vi "Dashboard Main.vi"() -> ()   [LabVIEW 2014]
uses:
  <vilib>/event_ctls.llb/eventvkey.ctl
  <vilib>/Rock Robotics/WPI/Dashboard/WPI_DashboardLogging Global.vi
  <vilib>/Rock Robotics/Network Tables/SD Write String.vi
  <vilib>/Rock Robotics/Network Tables/SD Write Numeric Array.vi
  <vilib>/Utility/config.llb/Write Key (String).vi
  <vilib>/Utility/config.llb/Write Key (I32).vi
  <vilib>/Utility/config.llb/NI_LVConfig.lvlib
panel:
  in  "Close Arm Time":dbl
  in  "TCP":refnum<k5>
  in  "Rec Mode":enum32{"Stop", "Record", "Playback"}(radio)
  in  "Vision":u16(ring) items=["Camera Off", "USB Camera SW", "USB Camera HW", "IP Camera"]
  out "Camera IP":string
  out "Image Message":string="Timeout in Camera Communications"
  in  "Dashboard Tab":T1(tab)
  in  "Camera Settings":T2={"Frame Rate"=30, "Compression"=30, "Size"=1} {"Frame Rate" scale=1.0..30.0; "Size" items=["640x480", "320x240", "160x120"]}
  out "MotorChart R":cluster{"Numeric":dbl, "Numeric":dbl}(graph)
  out "MotorChart L":T3(graph)
  out "MotorSliders R":cluster{"MotorSlide1":dbl, "MotorSlide2":dbl} {"MotorSlide2" scale=-1.0..1.0 scale format="%#_2e"; "MotorSlide1" scale=-1.0..1.0 scale format="%#_2e"}
  out "MotorSliders L":T4 {"MotorSlide4 2" scale=0.0..14.0 scale format="%#_2e"; "MotorSlide2" scale=-1.0..1.0 scale format="%#_2e"; "MotorSlide1" scale=-1.0..1.0 scale format="%#_2e"}
  out "Gyro":dbl(knob) scale=0.0..360.0
  out "JS1 Z":dbl(slide) scale=-1.0..1.0 scale format="%#_2e"
  out "JS1 Graph":cluster{"X":dbl, "Y":dbl}[](graph)
  out "JS1 Buttons":T5
  out "JS2 Z":dbl(slide) scale=-1.0..1.0 scale format="%#_2e"
  out "JS2 Graph":cluster{"X":dbl, "Y":dbl}[](graph)
  out "JS2 Buttons":T5
  out "Mode":T6(ring)=enum."Auto Disabled"
  in  "DB Camera Config":bool
  out "fps":dbl format="%#.1g"
  out "Mbps":dbl format="%#.1g"
  out "Mbps 2":bool
  in  "DB/String 9":string
  in  "DB/String 8":string
  in  "DB/String 7":string
  in  "DB/String 6":string
  in  "DB/String 5":string
  in  "DB/String 4":string
  in  "DB/String 3":string
  in  "DB/String 2":string
  in  "DB/String 1":string
  in  "DB/String 0":string
  in  "DB/Slider 0":dbl(slide) scale=0.0..5.0
  in  "DB/Slider 1":dbl(slide) scale=0.0..5.0
  in  "DB/Slider 2":dbl(slide) scale=0.0..5.0
  in  "DB/Slider 3":dbl(slide) scale=0.0..5.0
  out "DB/LED 3":bool
  out "DB/LED 2":bool
  out "DB/LED 1":bool
  out "DB/LED 0":bool
  in  "DB/Button 3":bool
  in  "DB/Button 2":bool
  in  "DB/Button 1":bool
  in  "DB/Button 0":bool caption="New Name"
  in  "Auto Mode":string(combo)
  in  "Slidewheel Speed":dbl
  in  "Desired Arm Speed":dbl
  in  "Drive Speed":dbl
  in  "Desired Arm Stop":dbl
  in  "Desired Stop Distance":dbl
  in  "Test Slider":dbl(slide) scale=0.0..100.0 scale format="%#_3g"
  in  "On/Off":bool caption="Solenoid"
  in  "Test Name":u16(ring) items=["Select the test to run...", "Example Test", "-------------------------------", "List of tests is built in robot code.", "Replace with your own automated tests."]
  in  "Test Tree":string(tree)
  in  "Motor":cluster{"Value":dbl, "Enable":bool} {"Value" scale=-1.0..1.0 scale format="%#_3g"}
  out "Progress":T7 {"Test Progress" scale=0.0..100.0}
  in  "Rev/Fwd":cluster{"Forward":bool, "Reverse":bool}
  in  "Test Ring":u16(ring) items=["Monochrome", "Color"]
  in  "Listbox":i32(listbox)
  out "Tree":string(tree)
  out "Camera Image":T8(plugin-control)
  out "Boolean":bool
  # "Left"
  # "Front"
  # "Right"
  # "Battery"
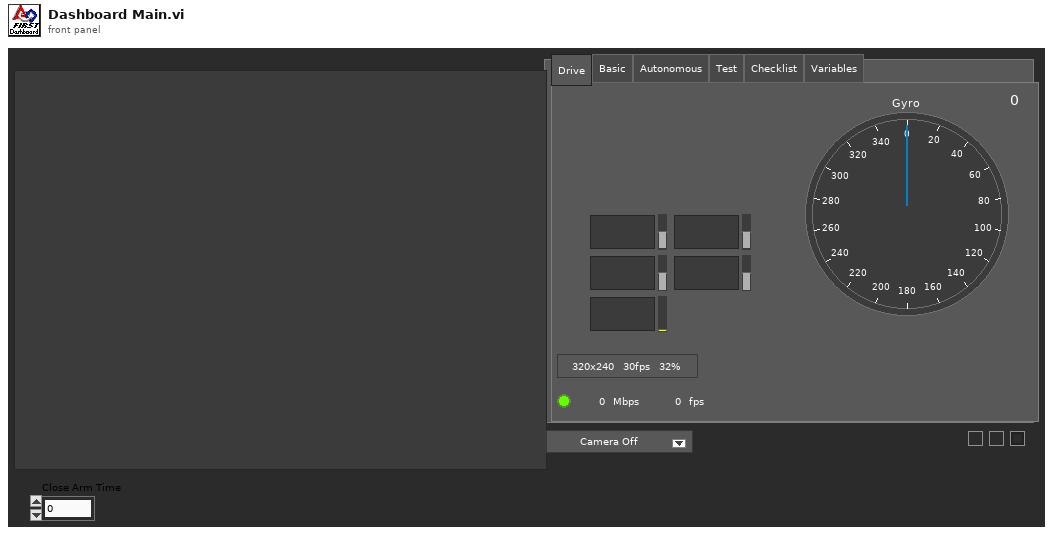
[diagram p1: front panel]
types:
  T1 = enum32{"Drive", "Basic", "Autonomous", "Test", "Checklist", "Variables"}
  T2 = cluster{"Frame Rate":i32, "Compression":i32, "Size":u16}
  T3 = cluster{"Numeric":dbl, "Numeric":dbl, "Battery V":dbl}
  T4 = cluster{"MotorSlide1":dbl, "MotorSlide2":dbl, "MotorSlide4 2":dbl}
  T5 = cluster{bool, bool, bool, bool, bool, bool, bool, bool, bool, bool, bool, bool}
  T6 = enum8{"Tele-Op Disabled", "Tele-Op Enabled", "Auto Disabled", "Auto Enabled", "Test Disabled", "Test Enabled", "Disconnected", "No Code", "E-Stop"}
  T7 = cluster{"Test Progress":u8, "Test Progress Text":string}
  T8 = typedef "IMAQ Image.ctl" = refnum<image>
  T9 = enum32{"Drive", "Basic", "Custom", "Test", "Checklist", "Variables"}
  T10 = typedef "Image Type" = u32
  T11 = cluster{"Camera Image":refnum<vi>, "Dashboard Tab":refnum<vi>, "Boolean":refnum<vi>, "Vision":refnum<vi>, "Rec Mode":refnum<vi>, "Test Slider":refnum<vi>, "On/Off ":refnum<vi>, "Test Ring":refnum<vi>, "Rev/Fwd":refnum<vi>, "Test Name":refnum<vi>, "Motor":refnum<vi>, "Progress":refnum<vi>, "CheckList":refnum<vi>, "Tree":refnum<vi>, "Test Tree":refnum<vi>}
  T12 = cluster{"Error Strings":string, "Disable Counts":cluster{u16, u16}, "Rail Faults":cluster{u16, u16, u16}, "Robot IP":string, "DB Mode":u8, "Event Info":cluster{"Name":string, "Type":u8, "Number":u16, "Replay":u8}, "Camera Addr":string}
  T13 = cluster{"Storage":cluster{"Disk Free":u64, "RAM Block":u32, "RAM free":u32}, "CPU Utilization":cluster{"CPU % ISR":sgl, "CPU % Time Crit":sgl, "CPU % Timed Str":sgl, "CPU % High":sgl, "CPU % Above":sgl, "CPU % Normal":sgl, "CPU % Low":sgl}, "CAN":cluster{"% Bus Utilization":sgl, "Bus Off Cnt":u32, "TX_FIFO Full Cnt":u32, "Receive Error Cnt":u8, "Transmit Error Cnt":u8}, "HID":cluster{"HID Outputs":u32, "Rumble Low":u16, "Rumble High":u16}[]}
  T14 = cluster{"Status bits":cluster{"Test Mode":bool, "Autonomous":bool, "Enabled":bool, "Code Start":bool, "Brownout":bool, "Reserved 2":bool, "Reserved 3":bool, "E-Stop":bool}, "Code Trace":cluster{"Disabled":bool, "TeleOp":bool, "Auto":bool, "Test":bool}, "Controller Type":enum16{"unknown", "cRIO", "roboRio"}, "Code?":enum16{"unknown", "noCode", "code"}, "Battery V":dbl}
  T15 = cluster{"Control Bits":cluster{"TestMode":bool, "Autonomous":bool, "Enabled":bool, "FMS Present":bool, bool, bool, bool, "E-Stop":bool}, "Team Station ":u8, "Countdown":sgl, "Joystick Values":cluster{"Axes":dbl[], "Buttons":bool[], "POVs":i16[]}[]}
  T16 = cluster{"Axes":dbl[], "Buttons":bool[], "POVs":i16[]}[]
  T17 = cluster{"Axes":dbl[], "Buttons":bool[], "POVs":i16[]}
  T18 = cluster{"Buttons[0]":bool, "Buttons[1]":bool, "Buttons[2]":bool, "Buttons[3]":bool, "Buttons[4]":bool, "Buttons[5]":bool, "Buttons[6]":bool, "Buttons[7]":bool, "Buttons[8]":bool, "Buttons[9]":bool, "Buttons[10]":bool, "Buttons[11]":bool}
  T19 = typedef "NI_LVConfig.lvlib/Config Data RefNum.ctl" = refnum<k1>
  T20 = cluster{"Operation":enum16{"Update", "Clear"}, "Color Box":u32}[]
  T21 = typedef "eventvkey.ctl" = enum16{"ASCII", "Enter", "Return", "Shift", "Ctrl", "Alt", "Cmd", "Opt", "Caps", "NumLock", "Clear", "Break", "Up", "Down", "Left", "Right", "Insert", "Delete", "Home", "End", "PageUp", "PageDown", "Escape", "Help", "Pause", "ScrollLock", "F1", "F2", "F3", "F4", "F5", "F6", "F7", "F8", "F9", "F10", "F11", "F12", "F13", "F14", "F15", "F16", "F17", "F18", "F19", "F20", "F21", "F22", "F23", "F24", "Play", "VolumeUp", "VolumeDown", "Mute", "Two Byte Char"}
  T22 = cluster{"Image Size":bool, "Image Type":bool, "Pixel Value":bool, "ROI Information":bool, "Zoom Factor":bool}
  T23 = enum8{"Enabled", "Disabled", "Disabled and Grayed Out"}
  T24 = cluster{"Operation":enum16{"Update", "Clear"}, "Color Box":u32}
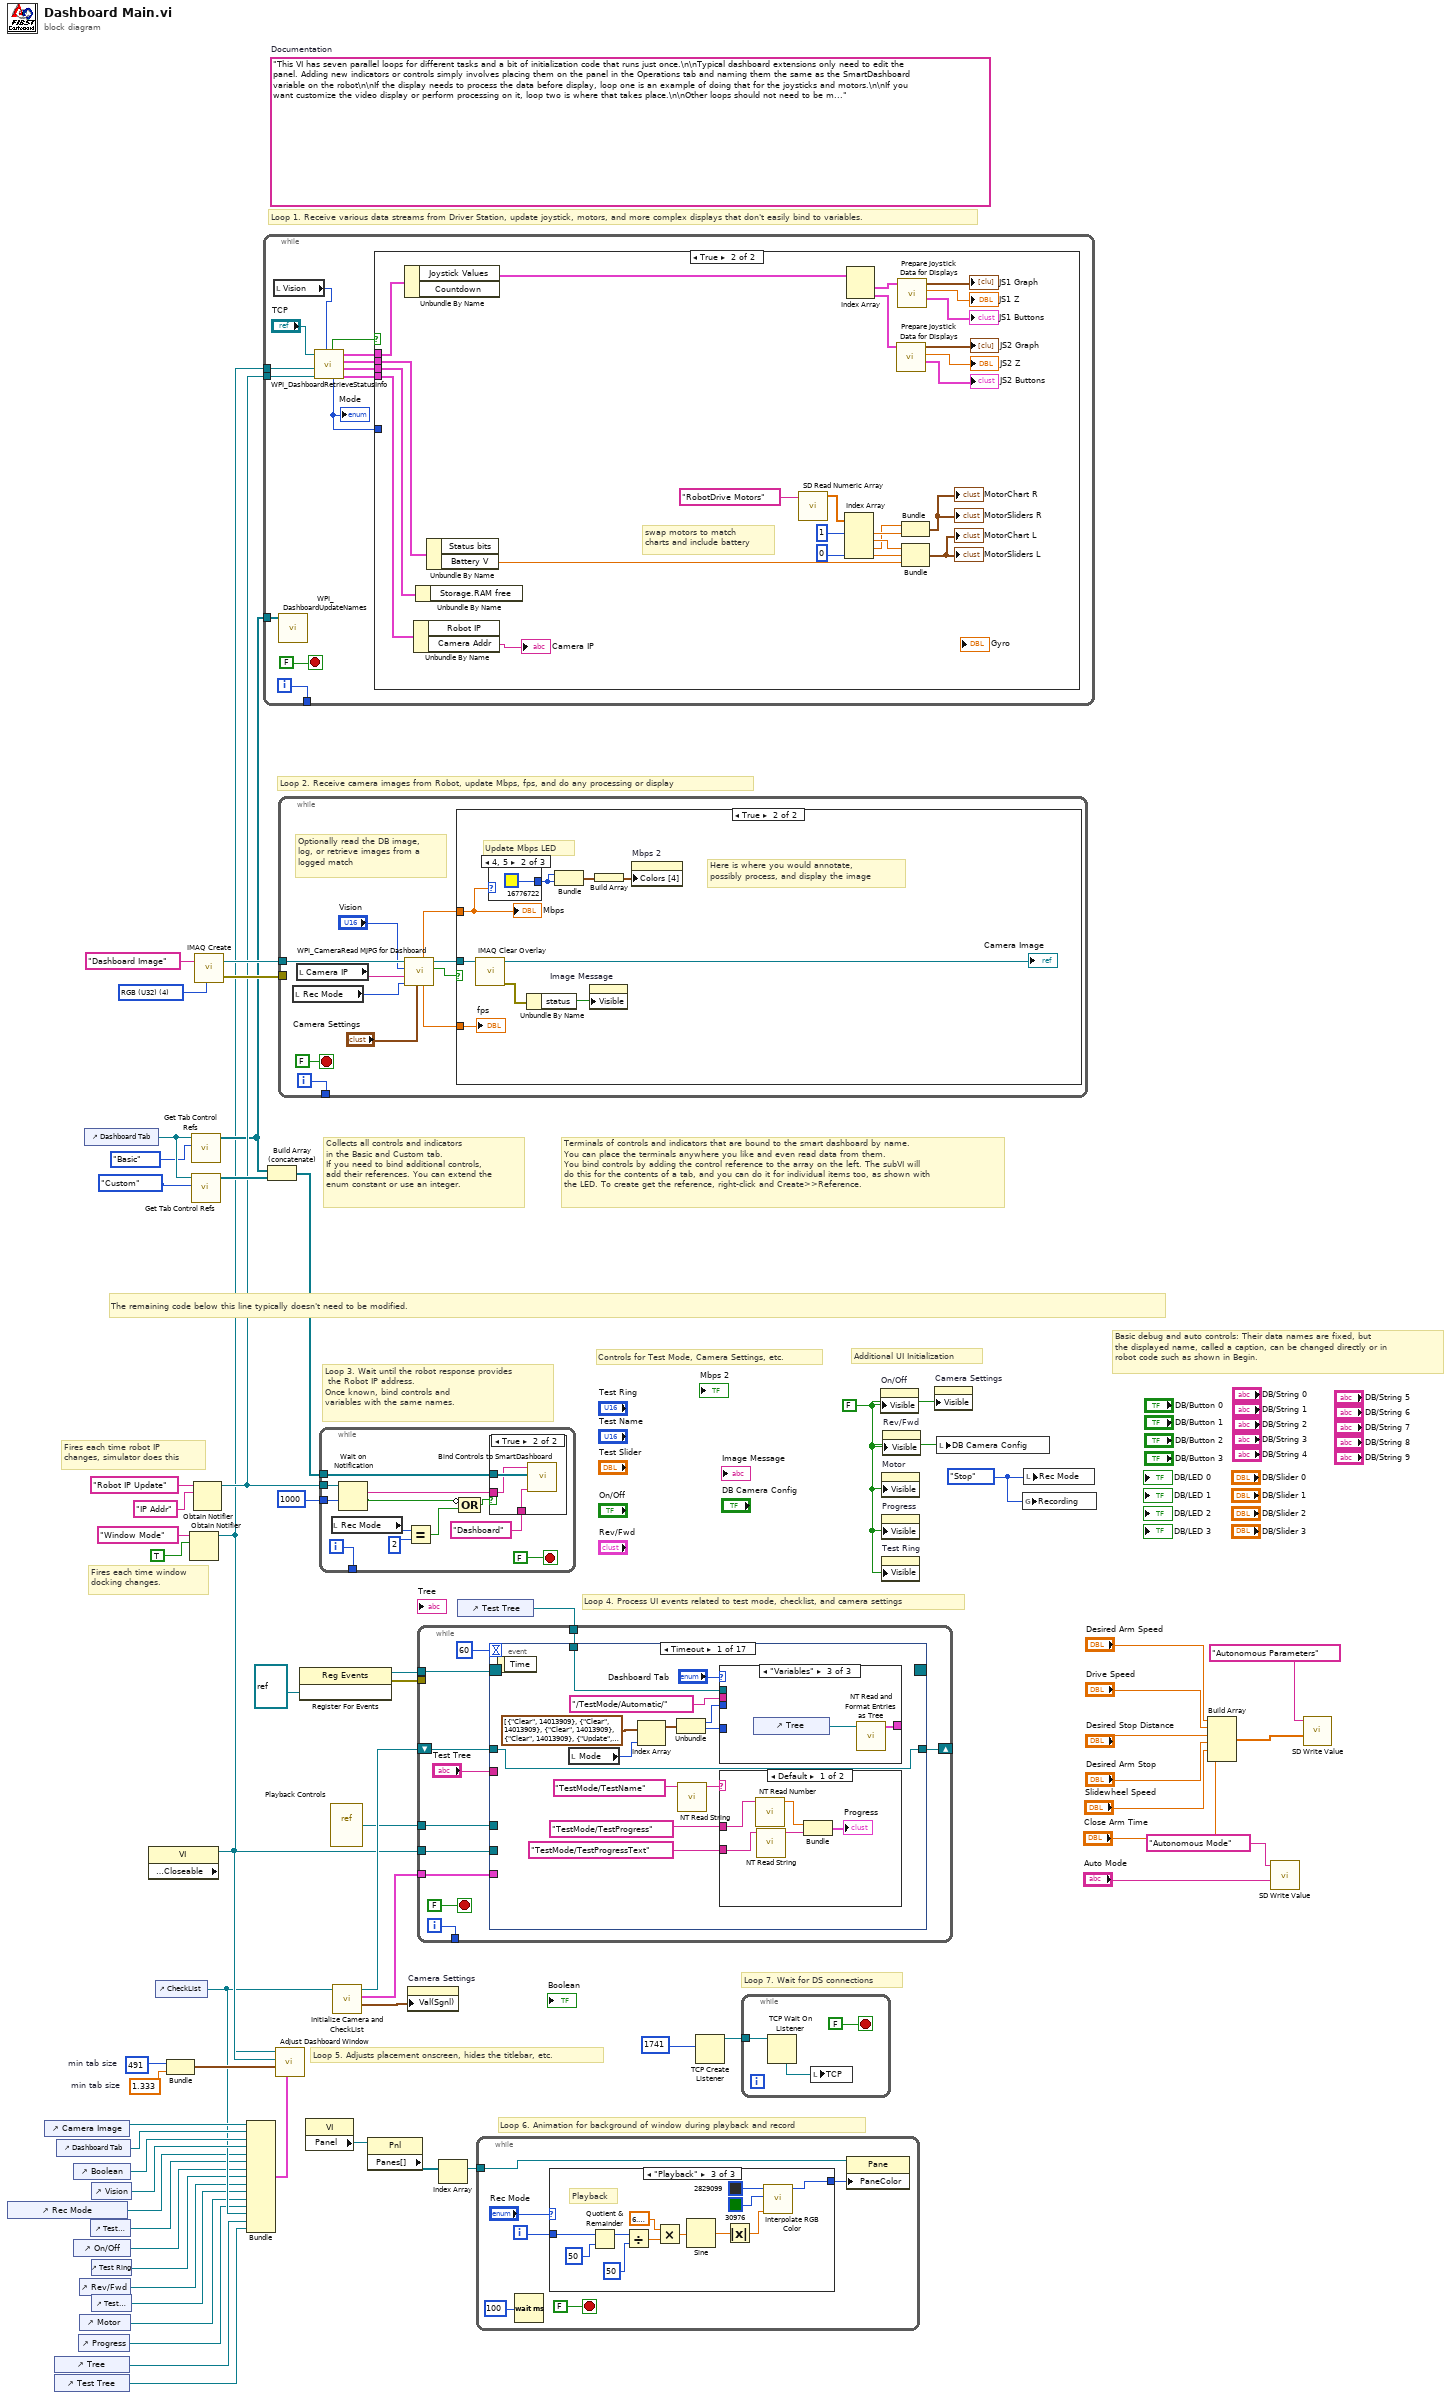
[diagram p0: block diagram]
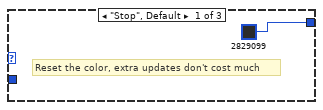
[diagram p3: hidden frame]
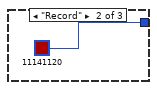
[diagram p4: hidden frame]
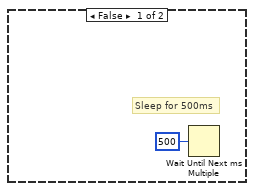
[diagram p6: hidden frame]
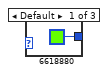
[diagram p7: hidden frame]
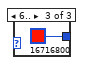
[diagram p8: hidden frame]
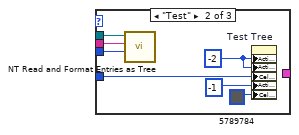
[diagram p10: hidden frame]
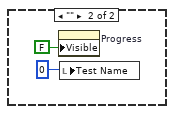
[diagram p11: hidden frame]
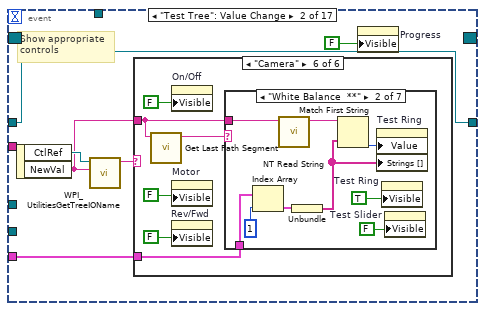
[diagram p12: hidden frame]
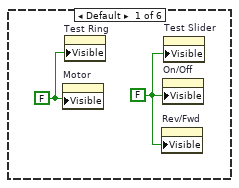
[diagram p13: hidden frame]
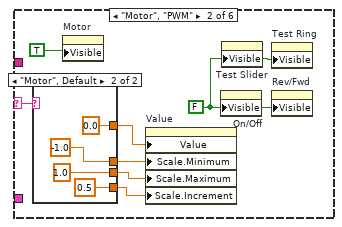
[diagram p14: hidden frame]
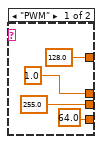
[diagram p15: hidden frame]
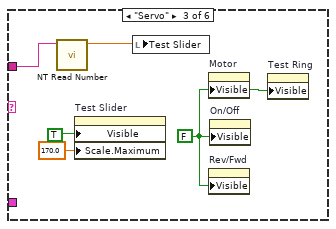
[diagram p16: hidden frame]
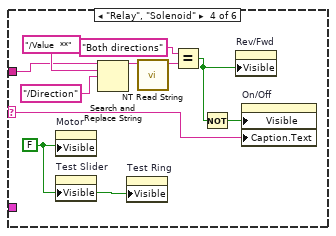
[diagram p17: hidden frame]
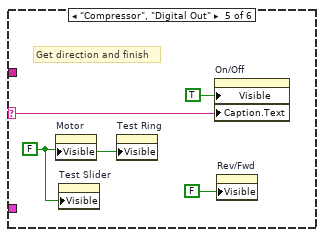
[diagram p18: hidden frame]
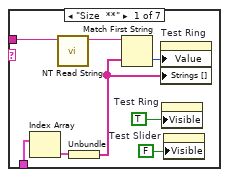
[diagram p19: hidden frame]
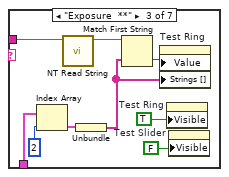
[diagram p20: hidden frame]
diagram:
  w34 = 491  # min tab size
  w33 = 1.333  # min tab size
  w42 = enum32{"Stop", "Record", "Playback"}."Stop" ("Rec Mode")
  w16 = FALSE ("Visible")
  (unwired) "This VI has seven parallel loops for different tasks and a bit of initialization code that runs just once.\n\nTypical dashboard extensions only need to edit the panel. Adding new indicators or controls simply involves placing them on the panel in the Operations tab and naming them the same as the SmartDashboard variable on the robot\n\nIf the display needs to process the data before display, loop one is an example of doing that for the joysticks and motors.\n\nIf you want customize the video display or perform processing on it, loop two is where that takes place.\n\nOther loops should not need to be modified. They are pretty standard, and document the task they perform."  # Documentation
  w62 = T10 4 items=["Grayscale (U8)", "Grayscale (I16)", "Grayscale (SGL)", "Complex (CSG)", "RGB (U32)", "HSL (U32)", "RGB (U64)"] ("Image Type")
  # "Loop 7. Wait for DS connections"
  # "Basic debug and auto controls: Their data names are fixed, but\nthe displayed name, called a caption, can be changed directly or in\nrobot code such as shown in Begin."
  # "Controls for Test Mode, Camera Settings, etc."
  # "Additional UI Initialization"
  # "Loop 6. Animation for background of window during playback and record"
  # "Fires each time robot IP\nchanges, simulator does this"
  # "Fires each time window\ndocking changes."
  # "Collects all controls and indicators\nin the Basic and Custom tab.\nIf you need to bind additional controls,\nadd their references. You can extend the\nenum constant or use an integer."
  # "The remaining code below this line typically doesn't need to be modified."
  # "Loop 4. Process UI events related to test mode, checklist, and camera settings"
  # "Terminals of controls and indicators that are bound to the smart dashboard by name.\nYou can place the terminals anywhere you like and even read data from them.\nYou bind controls by adding the control reference to the array on the left. The subVI will\ndo this for the contents of a tab, and you can do it for individual items too, as shown with\nthe LED. To create get the reference, right-click and Create>>Reference."
  # "Loop 3. Wait until the robot response provides\n the Robot IP address.\nOnce known, bind controls and\nvariables with the same names."
  # "Loop 5. Adjusts placement onscreen, hides the titlebar, etc."
  # "Loop 1. Receive various data streams from Driver Station, update joystick, motors, and more complex displays that don't easily bind to variables."
  # "Loop 2. Receive camera images from Robot, update Mbps, fps, and do any processing or display"
  n1 = control-ref of="Rec Mode"() -> (w22:refnum<vi>)
  n2 = control-ref of="Camera Image"() -> (w37:refnum<vi>)
  n3 = control-ref of="Tree"() -> (w26:refnum<vi>)
  n4 = control-ref of="Test Tree"() -> (w25:refnum<vi>)
  n5 = control-ref of="Dashboard Tab"() -> (w36:refnum<vi>)
  n6 = control-ref of="Boolean"() -> (w31:refnum<vi>)
  n7 = control-ref of="On/Off"() -> (w20:refnum<vi>)
  n8 = control-ref of="Progress"() -> (w17:refnum<vi>)
  n9 = control-ref of="Rev/Fwd"() -> (w18:refnum<vi>)
  n10 = control-ref of="Motor"() -> (w23:refnum<vi>)
  n11 = control-ref of="Dashboard Tab"() -> (w40:refnum<vi>)
  n12 = control-ref of="Test Slider"() -> (w21:refnum<vi>)
  n13 = control-ref of="Vision"() -> (w35:refnum<vi>)
  n14 = control-ref of="Test Ring"() -> (w19:refnum<vi>)
  n15 = control-ref of="Test Name"() -> (w24:refnum<vi>)
  n16 = property class="VI" props=["Front Panel.Closeable"]() -> (reference out=w41:refnum<vi>)  [unwired: 2 in, 2 out]
  n17 = control-ref of="CheckList"() -> (w27:refnum<vi>)
  n18 = Bundle("min tab size"=w34, "min tab size"=w33) -> (w32:cluster{"min tab size":i32, "min tab size":dbl})  [unwired: 1 in]
  n19 = Obtain Notifier(name (unnamed)="Window Mode", notification data type=TRUE) -> (notifier out=w13:refnum<notifier>)  [unwired: 2 in, 2 out]
  n20 = call <vilib>:"Get Tab Control Refs.vi"("Page Index"=T9."Basic" ("Dashboard Tab"), "TabControl in"=w40) -> ("ControlsOnPage"=w14:refnum<vi>[])  [unwired: 9 in]
  n21 = call <vilib>:"Get Tab Control Refs.vi"("Page Index"=T9."Custom" ("Dashboard Tab"), "TabControl in"=w40) -> ("ControlsOnPage"=w39:refnum<vi>[])  [unwired: 9 in]
  n22 = Obtain Notifier(name (unnamed)="Robot IP Update", notification data type="IP Addr" ("name (unnamed)")) -> (notifier out=w15:refnum<notifier>)  [unwired: 2 in, 2 out]
  n23 = call "IMAQ Create"("Image Name"="Dashboard Image", "Image Type"=w62) -> ("New Image"=w60:T8, "error out"=w59:errorcluster)  [unwired: 2 in, 1 out]
  n24 = Bundle("Camera Image"=w37, "Dashboard Tab"=w36, "Boolean"=w31, "Vision"=w35, "Rec Mode"=w22, "Test Slider"=w21, "On/Off"=w20, "Test Ring"=w19, "Rev/Fwd"=w18, "Test Name"=w24, "Motor"=w23, "Progress"=w17, "CheckList"=w27, "Tree"=w26, "Test Tree"=w25) -> (w28:T11)  [unwired: 1 in]
  n25 = while {
    tunnel: [w74] -> _
    tunnel: w15 -> [w68]
    tunnel: w14 -> [w67]
    tunnel: w13 -> [w63]
    i -> [w74]
    stop <- FALSE stop-if-true
    n26 = local read "Vision"() -> (w65:u16)
    n27 = call <vilib>:"WPI_DashboardUpdateNames.vi"("Controls on Tab"=w67) -> ()  [unwired: 11 in]
    n28 = call <vilib>:"WPI_DashboardRetrieveStatusInfo.vi"("Vision"=w65, "Binding Refnum"=w68, "Window Mode Notifier"=w63, "TCP Cnx"="TCP") -> ("Power and Errors"=w69:T12, "Robot Metrics"=w72:T13, "Status Info"=w73:T14, "Control Info"=w70:T15, "Robot Mode"=w66:T6, "Process?"=w71:bool)  [unwired: 2 in]
    "Mode" <- w66
    n29 = case shown="True" w71 {
      tunnel: w73 -> [_ w100]
      tunnel: w72 -> [_ w99]
      tunnel: w70 -> [_ w98]
      tunnel: w69 -> [_ w97]
      tunnel: w66 -> [_ _]
      frame False {
      }
      frame True {
        # "swap motors to match\ncharts and include battery"
        n30 = Unbundle By Name(w98) -> ("Joystick Values"=w85:T16)  [unwired: 1 out]
        n31 = Unbundle By Name(w97) -> ("Camera Addr"=→"Camera IP":string)  [unwired: 1 out]
        n32 = Unbundle By Name(w99) -> ()  [unwired: 1 out]
        n33 = Unbundle By Name(w100) -> ("Battery V"=w86:dbl)  [unwired: 1 out]
        n34 = call <vilib>:"SD Read Numeric Array.vi"("Name"="RobotDrive Motors") -> ("Numeric Array"=w88:dbl[])  [unwired: 8 in, 2 out]
        n35 = Index Array(array=w88, index #1=1, index #4=0) -> (element #1=w92:dbl, element #2=w93:dbl, element #3=w91:dbl, element #4=w96:dbl)  [unwired: 2 in]
        n36 = Index Array(array=w85) -> (element #1=w84:T17, element #2=w79:T17)  [unwired: 2 in]
        n37 = call "Prepare Joystick Data for Displays.vi"("Joystick Values"=w79) -> ("Buttons"=→"JS2 Buttons":T18, "Z Axis"=→"JS2 Z":dbl, "Cartesian Data"=→"JS2 Graph":cluster{"X axis":dbl, "X axis":dbl}[])  [unwired: 8 in]
        n38 = call "Prepare Joystick Data for Displays.vi"("Joystick Values"=w84) -> ("Buttons"=→"JS1 Buttons":T18, "Z Axis"=→"JS1 Z":dbl, "Cartesian Data"=→"JS1 Graph":cluster{"X axis":dbl, "X axis":dbl}[])  [unwired: 8 in]
        n39 = Bundle("Numeric"=w91, "Numeric"=w92) -> (→"MotorChart R" →"MotorSliders R":cluster{"Numeric":dbl, "Numeric":dbl})  [unwired: 1 in]
        n40 = Bundle("Numeric"=w93, "Numeric"=w96, "Battery V"=w86) -> (→"MotorChart L" →"MotorSliders L":T3)  [unwired: 1 in]
      }
    }
  }
  n41 = Build Array (concatenate)(w14, w39) -> (w38:refnum<vi>[])
  n42 = call "Adjust Dashboard Window.vi"("Sizing Refnums"=w28, "Size Constraints"=w32, "VI"=w41, "Notifier in"=w13) -> ()  [unwired: 8 in]
  n43 = while {
    tunnel: w60 -> [w109]
    tunnel: w59 -> [_]
    tunnel: [w110] -> _
    i -> [w110]
    stop <- FALSE stop-if-true
    # "Optionally read the DB image,\nlog, or retrieve images from a\nlogged match"
    n44 = local read "Rec Mode"() -> (w103:enum32{"Stop", "Record", "Playback"})
    n45 = local read "Camera IP"() -> (w101:string)
    n46 = call <vilib>:"WPI_CameraRead MJPG for Dashboard.vi"("Camera Settings"="Camera Settings", "Rec Mode"=w103, "Camera IP"=w101, "Camera Mode"="Vision", "Refnum in"=w109) -> ("Active"=w107:bool, "Refnum out"=w108:T8, "FPS"=w106:dbl, "Bandwidth (Mbps)"=w105:dbl)  [unwired: 3 in]
    n47 = case shown="True" w107 {
      tunnel: w108 -> [_ w116]
      tunnel: w105 -> [_ w115]
      tunnel: w106 -> [_ w113]
      frame False {
        # "Sleep for 500ms"
        n48 = Wait Until Next ms Multiple(millisecond multiple=u32 500) -> ()  [unwired: 1 out]
      }
      frame True {
        # "Here is where you would annotate,\npossibly process, and display the image"
        # "Update Mbps LED"
        n49 = call "IMAQ Clear Overlay"("Image"=w116) -> ("error out"=w120:errorcluster, "Image Out"=→"Camera Image":T8)  [unwired: 2 in, 7 out]
        n50 = case shown="4, 5" w115 {
          tunnel: [u32 6618880 ("Color Box") u32 16776722 ("Color Box") u32 16716800 ("Color Box")] -> w117
          frame Default {
          }
          frame 4, 5 {
          }
          frame 6.. {
          }
        }
        n51 = Unbundle By Name(w120) -> ("status"=w121:bool)
        n52 = Bundle("Color Box"=w117, "Color Box"=w117) -> (w119:cluster{"Color Box":u32, "Color Box":u32})  [unwired: 1 out]
        n53 = property on="Image Message" class="Str"("Visible"=w121) -> ()  [unwired: 2 in, 2 out]
        n54 = Build Array(w119) -> (w118:cluster{"Color Box":u32, "Color Box":u32}[])
        n55 = property on="Mbps 2" class="Bool (strict)"("Colors [4]"=w118) -> ()  [unwired: 2 in, 2 out]
        "Mbps" <- w115
        "fps" <- w113
      }
    }
  }
  n56 = register-events(refnum<vi> refnum) -> (reference out=w46:refnum<event-registration>, error out=w45:errorcluster)  [unwired: 2 in]
  n57 = property class="VI"() -> ("Panel"=w49:refnum<vi>)  [unwired: 2 in, 2 out]
  n58 = while {
    tunnel: w38 -> [w136]
    tunnel: w15 -> [w134]
    tunnel: [w132] -> _
    tunnel: u32 1000 ("milliseconds to wait") -> [w131]
    i -> [w132]
    stop <- FALSE stop-if-true
    n59 = local read "Rec Mode"() -> (w127:enum32{"Stop", "Record", "Playback"})
    n60 = Wait on Notification(notifier=w134, timeout in ms (-1)=w131) -> (notification=w133:string, timed out?=w129:bool)  [unwired: 2 in, 2 out]
    n61 = Equal?(x=w127, y=u16 2 ("Rec Mode")) -> (x = y?=w128:bool)
    n62 = Compound Arithmetic op=OR(invert w129, w128) -> (w130:bool)
    n63 = case shown="True" w130 {
      tunnel: w136 -> [_ w139]
      tunnel: w133 -> [_ w138]
      tunnel: "Dashboard" -> [_ w137]
      frame False {
      }
      frame True {
        n64 = call <vilib>:"Bind Controls to SmartDashboard.vi"("Client Name"=w137, "Bound Control Refs"=w139, "Server IP Address"=w138) -> ()  [unwired: 9 in]
      }
    }
  }
  n65 = vi-ref "Playback Controls.vi"() -> (w47:refnum<vi>)
  n66 = call "Initialize Camera and CheckList.vi"("ListBox in"=w27) -> ("Cluster"=w53:cluster{"value":i32, "value":i32, "index":i32}, "Array"=w54:cluster{string[]}[], "File Refnum"=w52:T19)  [unwired: 8 in]
  n67 = property class="Pnl"(reference=w49) -> ("Panes[]"=w50:refnum<vi>[])  [unwired: 1 in, 2 out]
  n68 = property on="Camera Settings" class="Clust (strict)"("Val(Sgnl)"=w53) -> ()  [unwired: 2 in, 2 out]
  n69 = Index Array(array=w50) -> (element=w48:refnum<vi>)  [unwired: 1 in]
  n70 = control-ref of="Test Tree"() -> (w51:refnum<vi>)
  n71 = while {
    tunnel: w54 -> [w147]
    shift-right: [w146] -> _
    shift-left: w52 -> [w145]
    tunnel: [w144] -> _
    tunnel: w51 -> [w143]
    tunnel: w47 -> [w142]
    tunnel: w46 -> [w141]
    tunnel: w45 -> [_]
    tunnel: w41 -> [w140]
    i -> [w144]
    stop <- FALSE stop-if-true
    n72 = event shown="[0] Timeout" {
      selector: w141 -> [_ _ _ _ _ _ _ _ _ _ _ _ _ _ _ _ _]
      dyn-events: [_ _ _ _ _ _ _ _ _ _ _ _ _ w385 _ _ _] -> _
      timeout: u32 60 ("milliseconds to wait") -> [_ _ _ _ _ _ _ _ _ _ _ _ _ _ _ _ _]
      tunnel: w143 -> [w159 _ _ _ _ _ _ _ _ _ _ _ _ _ _ _ _]
      tunnel: "Test Tree" -> [_ _ _ _ _ _ _ _ w354 w362 w364 w368 w376 _ _ _ _]
      tunnel: w147 -> [_ w181 _ _ _ _ w318 w348 _ _ _ _ _ _ _ _ _]
      tunnel: [w155 w180 w279 w284 w292 w304 w317 w341 w353 w360 w363 w367 w375 w387 w401 w402 w412] -> w146
      tunnel: w145 -> [w155 w180 w279 w284 w292 w304 w316 w341 w353 w360 w363 w367 w375 w387 w401 w402 w412]
      tunnel: w142 -> [_ _ _ _ _ _ _ _ _ _ _ _ _ w388 _ w405 _]
      tunnel: w140 -> [_ _ _ _ _ _ _ _ _ _ _ _ _ w383 _ _ _]
      event Timeout {
        n73 = event-data() -> ()  [unwired: 1 in, 1 out]
        n74 = local read "Mode"() -> (w158:T6)
        n75 = Index Array(array=T20 [{"Operation"=enum."Clear", "Color Box"=14013909}, {"Operation"=enum."Clear", "Color Box"=14013909}, {"Operation"=enum."Clear", "Color Box"=14013909}, {"Operation"=enum."Clear", "Color Box"=14013909}, {"Operation"=enum."Update", "Color Box"=14013909}, {"Operation"=enum."Update", "Color Box"=16777215}, {"Operation"=enum."Clear", "Color Box"=14013909}, {"Operation"=enum."Clear", "Color Box"=14013909}, {"Operation"=enum."Clear", "Color Box"=14013909}], index=w158) -> (element=w153:T24)
        n76 = Unbundle(w153) -> ("Operation"=w152:enum16{"Update", "Clear"}, "Color Box"=w151:u32)
        n77 = call <vilib>:"NT Read String.vi"("Name"="TestMode/TestName") -> ("String"=w162:string)  [unwired: 9 in, 1 out]
        n78 = case shown="\"Variables\"" "Dashboard Tab" {
          tunnel: w159 -> [_ w170 _]
          tunnel: "/TestMode/Automatic/" ("Name Pattern") -> [_ w169 _]
          tunnel: w152 -> [_ w168 _]
          tunnel: [_ _ w172] -> _
          tunnel: w151 -> [_ w164 _]
          frame "Autonomous", Default {
          }
          frame "Test" {
            w167 = -2 ("Active Item:Row Number")
            n79 = call <vilib>:"NT Read and Format Entries as Tree.vi"("Operation"=w168, "Name Pattern"=w169, "Tree Refnum"=w170) -> ()  [unwired: 7 in, 2 out]
            n80 = property on="Test Tree" class="Tree (strict)"("Active Item Row Number"=w167, "ActiveColNum"=w167, "CellBG"=w164, "Active Item Row Number"=-1 ("Active Item:Row Number"), "CellBG"=u32 5789784 ("Color Box")) -> ()  [unwired: 2 in, 2 out]
          }
          frame "Variables" {
            n81 = control-ref of="Tree"() -> (w171:refnum<vi>)
            n82 = call <vilib>:"NT Read and Format Entries as Tree.vi"("Tree Refnum"=w171) -> ("Formatted Strings"=w172:cluster{"Name":string, "Value":string}[])  [unwired: 9 in, 1 out]
          }
        }
        n83 = case shown="Default" w162 {
          tunnel: "TestMode/TestProgress" ("Name") -> [w174 _]
          tunnel: "TestMode/TestProgressText" ("Name") -> [w173 _]
          frame Default {
            n84 = call <vilib>:"NT Read Number.vi"("Name"=w174) -> ("Numeric"=w175:dbl)  [unwired: 9 in, 1 out]
            n85 = call <vilib>:"NT Read String.vi"("Name"=w173) -> ("String"=w176:string)  [unwired: 9 in, 1 out]
            n86 = Bundle("Numeric"=w175, "String"=w176) -> (→"Progress":cluster{"Numeric":dbl, "String":string})  [unwired: 1 in]
          }
          frame "" {
            n87 = property on="Progress" class="Clust (strict)"("Visible"=FALSE) -> ()  [unwired: 2 in, 2 out]
            n88 = local write "Test Name"(u16 0) -> ()
          }
        }
      }
      event "Test Tree": Value Change {
        # "Show appropriate\ncontrols"
        n89 = event-data() -> ("CtlRef"=w184:refnum<vi>, "NewVal"=w182:string)  [unwired: 1 in]
        n90 = call <vilib>:"WPI_UtilitiesGetTreeIOName.vi"("NewVal"=w182, "TreeControl in"=w184) -> ("I/O Name"=w185:string)  [unwired: 9 in]
        n91 = case shown="\"Camera\"" w185 {
          selector: w185 -> [_ w192 _ w210 w219 _]
          tunnel: w182 -> [_ _ w207 w209 _ w226]
          tunnel: w181 -> [_ _ _ _ _ w225]
          frame Default {
            w187 = FALSE ("Visible")
            w186 = FALSE ("Visible")
            n92 = property on="Motor" class="Clust (strict)"("Visible"=w186) -> ()  [unwired: 2 in, 2 out]
            n93 = property on="Test Ring" class="Ring (strict)"("Visible"=w186) -> ()  [unwired: 2 in, 2 out]
            n94 = property on="Rev/Fwd" class="Clust (strict)"("Visible"=w187) -> ()  [unwired: 2 in, 2 out]
            n95 = property on="On/Off" class="Bool (strict)"("Visible"=w187) -> ()  [unwired: 2 in, 2 out]
            n96 = property on="Test Slider" class="Slide (strict)"("Visible"=w187) -> ()  [unwired: 2 in, 2 out]
          }
          frame "Motor", "PWM" {
            w193 = FALSE ("Visible")
            n97 = case shown="\"Motor\", Default" w192 {
              tunnel: [1.0 ("Value") -1.0 ("Value")] -> w191
              tunnel: [255.0 ("Value") 1.0 ("Value")] -> w190
              tunnel: [128.0 ("Value") 0.0 ("Value")] -> w189
              tunnel: [64.0 ("Value") 0.5 ("Value")] -> w188
              frame "PWM" {
              }
              frame "Motor", Default {
              }
            }
            n98 = property on="Motor" class="Clust (strict)"("Visible"=TRUE) -> ()  [unwired: 2 in, 2 out]
            n99 = property on="Value" class="Slide (strict)"("Value"=w189, "Scale.Minimum"=w191, "Scale.Maximum"=w190, "Scale.Increment"=w188) -> ()  [unwired: 2 in, 2 out]
            n100 = property on="On/Off" class="Bool (strict)"("Visible"=w193) -> ()  [unwired: 2 in, 2 out]
            n101 = property on="Test Slider" class="Slide (strict)"("Visible"=w193) -> ()  [unwired: 2 in, 2 out]
            n102 = property on="Test Ring" class="Ring (strict)"("Visible"=w193) -> ()  [unwired: 2 in, 2 out]
            n103 = property on="Rev/Fwd" class="Clust (strict)"("Visible"=w193) -> ()  [unwired: 2 in, 2 out]
          }
          frame "Servo" {
            w205 = FALSE ("Visible")
            n104 = call <vilib>:"NT Read Number.vi"("Name"=w207) -> ("Numeric"=w206:dbl)  [unwired: 9 in, 1 out]
            n105 = property on="Test Slider" class="Slide (strict)"("Visible"=TRUE, "Scale.Maximum"=170.0 ("Scale.Range:Maximum")) -> ()  [unwired: 2 in, 2 out]
            n106 = local write "Test Slider"(w206) -> ()
            n107 = property on="Motor" class="Clust (strict)"("Visible"=w205) -> ()  [unwired: 2 in, 2 out]
            n108 = property on="Rev/Fwd" class="Clust (strict)"("Visible"=w205) -> ()  [unwired: 2 in, 2 out]
            n109 = property on="On/Off" class="Bool (strict)"("Visible"=w205) -> ()  [unwired: 2 in, 2 out]
            n110 = property on="Test Ring" class="Ring (strict)"("Visible"=w205) -> ()  [unwired: 2 in, 2 out]
          }
          frame "Relay", "Solenoid" {
            w208 = FALSE ("Visible")
            n111 = property on="Motor" class="Clust (strict)"("Visible"=w208) -> ()  [unwired: 2 in, 2 out]
            n112 = property on="Test Slider" class="Slide (strict)"("Visible"=w208) -> ()  [unwired: 2 in, 2 out]
            n113 = Search and Replace String(input string=w209, search string="/Value  **", replace string="/Direction") -> (result string=w215:string)  [unwired: 5 in, 3 out]
            n114 = property on="Test Ring" class="Ring (strict)"("Visible"=w208) -> ()  [unwired: 2 in, 2 out]
            n115 = call <vilib>:"NT Read String.vi"("Name"=w215) -> ("String"=w213:string)  [unwired: 9 in, 1 out]
            n116 = Equal?(x="Both directions", y=w213) -> (x = y?=w211:bool)
            n117 = Not(x=w211) -> (.not. x?=w212:bool)
            n118 = property on="Rev/Fwd" class="Clust (strict)"("Visible"=w211) -> ()  [unwired: 2 in, 2 out]
            n119 = property on="On/Off" class="Bool (strict)"("Visible"=w212, "Caption.Text"=w210) -> ()  [unwired: 2 in, 2 out]
          }
          frame "Compressor", "Digital Out" {
            w218 = FALSE ("Visible")
            # "Get direction and finish"
            n120 = property on="Motor" class="Clust (strict)"("Visible"=w218) -> ()  [unwired: 2 in, 2 out]
            n121 = property on="Test Slider" class="Slide (strict)"("Visible"=w218) -> ()  [unwired: 2 in, 2 out]
            n122 = property on="Test Ring" class="Ring (strict)"("Visible"=w218) -> ()  [unwired: 2 in, 2 out]
            n123 = property on="On/Off" class="Bool (strict)"("Visible"=TRUE, "Caption.Text"=w219) -> ()  [unwired: 2 in, 2 out]
            n124 = property on="Rev/Fwd" class="Clust (strict)"("Visible"=FALSE) -> ()  [unwired: 2 in, 2 out]
          }
          frame "Camera" {
            n125 = call <vilib>:"Get Last Path Segment.vi"("String in"=w226) -> ("String out"=w227:string)  [unwired: 10 in]
            n126 = property on="On/Off" class="Bool (strict)"("Visible"=FALSE) -> ()  [unwired: 2 in, 2 out]
            n127 = property on="Motor" class="Clust (strict)"("Visible"=FALSE) -> ()  [unwired: 2 in, 2 out]
            n128 = property on="Rev/Fwd" class="Clust (strict)"("Visible"=FALSE) -> ()  [unwired: 2 in, 2 out]
            n129 = case shown="\"White Balance  **\"" w227 {
              tunnel: w226 -> [w233 w242 w251 w260 w269 _ w275]
              tunnel: w225 -> [w231 w239 w248 w257 w266 _ _]
              frame "Size  **" {
                n130 = Index Array(array=w231) -> (element=w230:cluster{string[]})  [unwired: 1 in]
                n131 = call <vilib>:"NT Read String.vi"("Name"=w233) -> ("String"=w232:string)  [unwired: 9 in, 1 out]
                n132 = Unbundle(w230) -> (w228:string[])
                n133 = Match First String(2:w228, 3:w232) -> (0:w229:i32)  [unwired: 1 out]
                n134 = property on="Test Ring" class="Ring (strict)"("Value"=w229, "Strings []"=w228) -> ()  [unwired: 2 in, 2 out]
                n135 = property on="Test Ring" class="Ring (strict)"("Visible"=TRUE) -> ()  [unwired: 2 in, 2 out]
                n136 = property on="Test Slider" class="Slide (strict)"("Visible"=FALSE) -> ()  [unwired: 2 in, 2 out]
              }
              frame "White Balance  **" {
                n137 = Index Array(array=w239, index=1) -> (element=w240:cluster{string[]})
                n138 = call <vilib>:"NT Read String.vi"("Name"=w242) -> ("String"=w241:string)  [unwired: 9 in, 1 out]
                n139 = Unbundle(w240) -> (w237:string[])
                n140 = Match First String(2:w237, 3:w241) -> (0:w236:i32)  [unwired: 1 out]
                n141 = property on="Test Ring" class="Ring (strict)"("Value"=w236, "Strings []"=w237) -> ()  [unwired: 2 in, 2 out]
                n142 = property on="Test Ring" class="Ring (strict)"("Visible"=TRUE) -> ()  [unwired: 2 in, 2 out]
                n143 = property on="Test Slider" class="Slide (strict)"("Visible"=FALSE) -> ()  [unwired: 2 in, 2 out]
              }
              frame "Exposure  **" {
                n144 = Index Array(array=w248, index=2) -> (element=w249:cluster{string[]})
                n145 = call <vilib>:"NT Read String.vi"("Name"=w251) -> ("String"=w250:string)  [unwired: 9 in, 1 out]
                n146 = Unbundle(w249) -> (w245:string[])
                n147 = Match First String(2:w245, 3:w250) -> (0:w246:i32)  [unwired: 1 out]
                n148 = property on="Test Ring" class="Ring (strict)"("Value"=w246, "Strings []"=w245) -> ()  [unwired: 2 in, 2 out]
                n149 = property on="Test Ring" class="Ring (strict)"("Visible"=TRUE) -> ()  [unwired: 2 in, 2 out]
                n150 = property on="Test Slider" class="Slide (strict)"("Visible"=FALSE) -> ()  [unwired: 2 in, 2 out]
              }
              frame "Exposure Priority  **" {
                n151 = Index Array(array=w257, index=3) -> (element=w258:cluster{string[]})
                n152 = call <vilib>:"NT Read String.vi"("Name"=w260) -> ("String"=w259:string)  [unwired: 9 in, 1 out]
                n153 = Unbundle(w258) -> (w254:string[])
                n154 = Match First String(2:w254, 3:w259) -> (0:w255:i32)  [unwired: 1 out]
                n155 = property on="Test Ring" class="Ring (strict)"("Value"=w255, "Strings []"=w254) -> ()  [unwired: 2 in, 2 out]
                n156 = property on="Test Ring" class="Ring (strict)"("Visible"=TRUE) -> ()  [unwired: 2 in, 2 out]
                n157 = property on="Test Slider" class="Slide (strict)"("Visible"=FALSE) -> ()  [unwired: 2 in, 2 out]
              }
              frame "Color Enable  **" {
                n158 = Index Array(array=w266, index=4) -> (element=w267:cluster{string[]})
                n159 = call <vilib>:"NT Read String.vi"("Name"=w269) -> ("String"=w268:string)  [unwired: 9 in, 1 out]
                n160 = Unbundle(w267) -> (w263:string[])
                n161 = Match First String(2:w263, 3:w268) -> (0:w264:i32)  [unwired: 1 out]
                n162 = property on="Test Ring" class="Ring (strict)"("Value"=w264, "Strings []"=w263) -> ()  [unwired: 2 in, 2 out]
                n163 = property on="Test Ring" class="Ring (strict)"("Visible"=TRUE) -> ()  [unwired: 2 in, 2 out]
                n164 = property on="Test Slider" class="Slide (strict)"("Visible"=FALSE) -> ()  [unwired: 2 in, 2 out]
              }
              frame Default {
                n165 = property on="Test Ring" class="Ring (strict)"("Visible"=FALSE) -> ()  [unwired: 2 in, 2 out]
                n166 = property on="Test Slider" class="Slide (strict)"("Visible"=FALSE) -> ()  [unwired: 2 in, 2 out]
              }
              frame "Brightness  **", "Color Level  **", "Compression  **", "FPS  **", "Sharpness  **" {
                n167 = call <vilib>:"NT Read Number.vi"("Name"=w275) -> ("Numeric"=w274:dbl)  [unwired: 9 in, 1 out]
                n168 = local write "Test Slider"(w274) -> ()
                n169 = property on="Test Slider" class="Slide (strict)"("Visible"=TRUE, "Scale.Maximum"=100.0 ("Scale.Range:Maximum")) -> ()  [unwired: 2 in, 2 out]
                n170 = property on="Test Ring" class="Ring (strict)"("Visible"=FALSE) -> ()  [unwired: 2 in, 2 out]
              }
            }
          }
        }
        n171 = property on="Progress" class="Clust (strict)"("Visible"=FALSE) -> ()  [unwired: 2 in, 2 out]
      }
      event "Test Name": Mouse Enter {
        # "Populate the ring with the list of tests"
        n172 = event-data() -> ()  [unwired: 1 in, 1 out]
        n173 = call <vilib>:"NT Read String Array.vi"("Name"="TestMode/TestList") -> ("String Array"=w283:string[])  [unwired: 9 in, 1 out]
        n174 = Build Array (concatenate)("Select the test to run...", w283) -> (w282:string[])
        n175 = property on="Test Name" class="Ring (strict)"("Strings []"=w282) -> ()  [unwired: 2 in, 2 out]
      }
      event "Test Name": Value Change {
        w285 = FALSE ("Visible")
        # "Tell the robot the test name to run"
        n176 = event-data() -> ("NewVal"=w289:u16)  [unwired: 1 in]
        n177 = property on="Test Name" class="Ring (strict)"() -> ("Strings []"=w290:string[])  [unwired: 2 in, 2 out]
        n178 = local write "Progress"(T7 {"Test Progress"=0, "Test Progress Text"=""} ("Progress")) -> ()
        n179 = Index Array(array=w290, index=w289) -> (element=w288:string)
        n180 = call <vilib>:"NT Write String.vi"("String"=w288, "Name"="TestMode/TestName") -> ()  [unwired: 9 in, 1 out]
        n181 = property on="Progress" class="Clust (strict)"("Visible"=TRUE) -> ()  [unwired: 2 in, 2 out]
        n182 = property on="Motor" class="Clust (strict)"("Visible"=w285) -> ()  [unwired: 2 in, 2 out]
        n183 = property on="Test Slider" class="Slide (strict)"("Visible"=w285) -> ()  [unwired: 2 in, 2 out]
        n184 = property on="On/Off" class="Bool (strict)"("Visible"=w285) -> ()  [unwired: 2 in, 2 out]
        n185 = property on="Rev/Fwd" class="Clust (strict)"("Visible"=w285) -> ()  [unwired: 2 in, 2 out]
        n186 = property on="Test Ring" class="Ring (strict)"("Visible"=w285) -> ()  [unwired: 2 in, 2 out]
      }
      event "Listbox": Double Click {
        # "Shift clears all"
        # "Update symbols on the listbox"
        n187 = event-data() -> ("PlatMods.Shift"=w293:bool, "Row"=w295:i32)  [unwired: 1 in]
        n188 = case shown="True" w293 {
          tunnel: w295 -> [w299 _]
          tunnel: 1 -> [w298 _]
          frame False {
            n189 = property on="Listbox" class="LstBox (strict)"() -> ("Item Symbols"=w297:i32[])  [unwired: 2 in, 2 out]
            n190 = Replace Array Subset(array=w297, new element=w298, index=w299) -> (w296:i32[])
            n191 = property on="Listbox" class="LstBox (strict)"("Item Symbols"=w296) -> ()  [unwired: 2 in, 2 out]
          }
          frame True {
            w300 = 0 ("Top Row")
            n192 = property on="Listbox" class="LstBox (strict)"() -> ("Number of Rows"=w302:u32)  [unwired: 2 in, 2 out]
            n193 = Initialize Array(0, w302) -> (w301:i32[])
            n194 = property on="Listbox" class="LstBox (strict)"("Top Row"=w300, "Value"=w300, "Item Symbols"=w301) -> ()  [unwired: 2 in, 2 out]
          }
        }
      }
      event "Listbox": Key Down {
        # "Update symbols on the listbox\nLeft and right keys check and uncheck"
        n195 = event-data() -> ("VKey"=w306:T21)  [unwired: 1 in]
        n196 = case shown="\"Left\", \"Right\"" w306 {
          selector: w306 -> [w311 _]
          tunnel: eventvkey."Left" ("VKey") -> [w309 _]
          frame "Left", "Right" {
            n197 = Equal?(x=w309, y=w311) -> (x = y?=w310:bool)
            n198 = Select(t=0, s=w310, f=1) -> (s? t:f=w312:i32)
            n199 = property on="Listbox" class="LstBox (strict)"() -> ("Item Symbols"=w315:i32[])  [unwired: 2 in, 2 out]
            n200 = Replace Array Subset(array=w315, new element=w312, index="Listbox") -> (w314:i32[])
            n201 = property on="Listbox" class="LstBox (strict)"("Item Symbols"=w314) -> ()  [unwired: 2 in, 2 out]
          }
          frame Default {
          }
        }
      }
      event "DB Camera Config": Value Change {
        # "Show or hide the cluster of controls, store in ini file"
        n202 = event-data() -> ("NewVal"=w319:bool)  [unwired: 1 in]
        n203 = case shown="False" w319 {
          tunnel: w318 -> [w328 _]
          tunnel: [w321 w339] -> w317
          tunnel: w316 -> [w320 w339]
          frame False {
            w335 = "Camera"
            w338 = FALSE ("Visible")
            n204 = local read "Camera Settings"() -> (w327:T2)
            n205 = Index Array(array=w328) -> (element=w331:cluster{string[]})  [unwired: 1 in]
            n206 = Unbundle(w327) -> ("Frame Rate"=w326:i32, "Compression"=w325:i32, "Size"=w329:u16)
            n207 = Unbundle(w331) -> (w330:string[])
            n208 = Index Array(array=w330, index=w329) -> (element=w324:string)
            n209 = call-poly <vilib>:"Write Key.vi"("section"=w335, "value"=w324, "key"="Size", "refnum"=w320) -> ("refnum out"=w337:T19)  [unwired: 2 in, 5 out]
            n210 = call-poly <vilib>:"Write Key.vi"("section"=w335, "value"=w326, "key"="FrameRate", "refnum"=w337) -> ("refnum out"=w336:T19)  [unwired: 1 in, 6 out]
            n211 = property on="Camera Settings" class="Clust (strict)"("Visible"=w338) -> ()  [unwired: 2 in, 2 out]
            n212 = local write "DB Camera Config"(w338) -> ()
            n213 = call-poly <vilib>:"Write Key.vi"("section"=w335, "value"=w325, "key"="Compression", "refnum"=w336) -> ("refnum out"=w322:T19)  [unwired: 1 in, 6 out]
            n214 = call <vilib>:"Close Config Data.vi"("refnum"=w322) -> ("file path"=w323:path)  [unwired: 2 in, 8 out]
            n215 = call <vilib>:"Open Config Data.vi"("configuration file path"=w323) -> ("refnum"=w321:T19)  [unwired: 8 in, 2 out]
          }
          frame True {
            n216 = property on="Camera Settings" class="Clust (strict)"("Visible"=TRUE) -> ()  [unwired: 2 in, 2 out]
          }
        }
      }
      event "Camera Settings": Value Change {
        # "Update summary string when any elements of DB camera change"
        n217 = event-data() -> ("NewVal"=w352:T2)  [unwired: 1 in]
        n218 = Index Array(array=w348) -> (element=w347:cluster{string[]})  [unwired: 1 in]
        n219 = Unbundle(w352) -> ("Frame Rate"=w343:i32, "Compression"=w342:i32, "Size"=w345:u16)
        n220 = Unbundle(w347) -> (w346:string[])
        n221 = Index Array(array=w346, index=w345) -> (element=w344:string)
        n222 = Format Into String(format string="%s   %dfps   %d%%", w344, w343, w342) -> (resulting string=w349:string)  [unwired: 2 in, 1 out]
        n223 = Build Array(w349) -> (w350:string[])
        n224 = property on="DB Camera Config" class="Bool (strict)"("Strings [4]"=w350) -> ()  [unwired: 2 in, 2 out]
      }
      event "Motor.Enable": Value Change {
        # "When the test mode otor enable helper is set, update that\ntree row item's value"
        n225 = event-data() -> ("NewVal"=w358:bool)  [unwired: 1 in]
        n226 = Unbundle("Motor") -> ("Value"=w357:dbl)  [unwired: 1 out]
        n227 = Select(t=w357, s=w358, f=0.0) -> (s? t:f=w355:dbl)
        n228 = call <vilib>:"NT Write Number.vi"("Numeric"=w355, "Name"=w354) -> ()  [unwired: 9 in, 1 out]
      }
      event "Test Slider": Value Change {
        # "When the test mode slider helper is set, update that\ntree row item's value"
        n229 = event-data() -> ("NewVal"=w361:dbl)  [unwired: 1 in]
        n230 = call <vilib>:"NT Write Number.vi"("Numeric"=w361, "Name"=w362) -> ()  [unwired: 9 in, 1 out]
      }
      event "On/Off": Value Change {
        # "When the test mode on/off helper value is set, update that\ntree row item's value"
        n231 = event-data() -> ("NewVal"=w366:bool)  [unwired: 1 in]
        n232 = Boolean To (0,1)(Boolean=w366) -> (0, 1=w365:i16)
        n233 = call <vilib>:"NT Write Number.vi"("Numeric"=w365, "Name"=w364) -> ()  [unwired: 9 in, 1 out]
      }
      event "Rev/Fwd": Value Change {
        # "When the test mode helper value for relays is set, update that\ntree row item's value"
        n234 = event-data() -> ("NewVal.Forward"=w374:bool, "NewVal.Reverse"=w373:bool)  [unwired: 1 in]
        n235 = Boolean To (0,1)(Boolean=w374) -> (0, 1=w370:i16)
        n236 = Boolean To (0,1)(Boolean=w373) -> (0, 1=w372:i16)
        n237 = Negate(x=w372) -> (-x=w371:i16)
        n238 = Add(x=w370, y=w371) -> (x+y=w369:i16)
        n239 = call <vilib>:"NT Write Number.vi"("Numeric"=w369, "Name"=w368) -> ()  [unwired: 9 in, 1 out]
      }
      event "Test Ring": Value Change {
        # "When a test mode helper value is selected from the ring,\nset the tree item's variable to the string value"
        n240 = event-data() -> ("NewVal"=w378:u16)  [unwired: 1 in]
        n241 = property on="Test Ring" class="Ring (strict)"() -> ("Strings []"=w379:string[])  [unwired: 2 in, 2 out]
        n242 = Index Array(array=w379, index=w378) -> (element=w377:string)
        n243 = call <vilib>:"NT Write String.vi"("String"=w377, "Name"=w376) -> ()  [unwired: 9 in, 1 out]
      }
      event "Rec Mode": Value Change {
        # "Update globals for recording mode and path to read log from.\nClear when logging and let NetworkTables set path for vision to\nuse."
        n244 = event-data() -> ("NewVal"=w389:enum32{"Stop", "Record", "Playback"})  [unwired: 1 in]
        n245 = global write "WPI_DashboardLogging Global.vi" "Logging Filename"(path "") -> ()
        n246 = case shown="\"Playback\"" w389 {
          tunnel: w388 -> [_ w391 w399]
          tunnel: [_ _ w398] -> w385
          tunnel: [_ _ w397] -> _
          tunnel: w383 -> [_ _ w395]
          tunnel: cluster{i32, i32} {-250, 170} -> [_ _ w394]
          tunnel: [_ _ T22 {"Image Size"=TRUE, "Image Type"=TRUE, "Pixel Value"=TRUE, "ROI Information"=TRUE, "Zoom Factor"=FALSE} ("Image Information Shown:All Elements")] -> w381
          tunnel: [_ _ TRUE ("Zoom Factor")] -> w380
          frame Default {
          }
          frame "Stop", "Record" {
            # "Place Window too"
            n247 = invoke class="VI" method="FP.Close"(reference=w391) -> (reference out=w390:refnum<vi>)  [unwired: 2 in, 2 out]
            n248 = invoke class="VI" method="Abort VI"(reference=w390) -> ()  [unwired: 2 in, 3 out]
          }
          frame "Playback" {
            n249 = call "Open Playback Panel.vi"("Offset"=w394, "DB VI Ref"=w395, "Playback in"=w399) -> ("Playback out"=w396:refnum<vi>)  [unwired: 8 in]
            n250 = register-events(w396) -> (reference out=w398:refnum<event-registration>, error out=w397:errorcluster)  [unwired: 2 in]
          }
        }
        n251 = global write "WPI_DashboardLogging Global.vi" "Recording"(w389) -> ()
        n252 = property on="Camera Image" class="ImageControl"("Image Information Shown"=w381, "Image Information Visible"=w380) -> ()  [unwired: 2 in, 2 out]
        n253 = call <vilib>:"WPI_DashboardNT Log FieldName Cache.vi"("Operation"=enum16{"Lookup/Add", "Index", "Clear"}."Clear") -> ()  [unwired: 8 in, 3 out]
      }
      event Panel Close {
        w400 = enum32{"Stop", "Record", "Playback"}."Stop" ("Rec Mode")
        # "Playback window has been closed, abort"
        n254 = event-data() -> ()  [unwired: 1 in, 4 out]
        n255 = local write "Rec Mode"(w400) -> ()
        n256 = global write "WPI_DashboardLogging Global.vi" "Recording"(w400) -> ()
      }
      event Panel Close {
        # "Abort playback window and ourself"
        n257 = event-data() -> ()  [unwired: 1 in, 4 out]
        n258 = invoke class="VI" method="FP.Close"(reference=w405) -> (reference out=w404:refnum<vi>)  [unwired: 2 in, 2 out]
        n259 = invoke class="VI" method="Abort VI"(reference=w404) -> (error out=w403:errorcluster)  [unwired: 2 in, 2 out]
        n260 = invoke class="VI" method="Abort VI"(error in=w403) -> ()  [unwired: 2 in, 3 out]
      }
      event "Vision": Value Change {
        # "Enable/Disable Compression slider.\nHW USB is hard-coded into the camera"
        n261 = event-data() -> ("NewVal"=w411:u16)  [unwired: 1 in]
        n262 = Equal?(x=w411, y=u32 2 ("milliseconds to wait")) -> (x = y?=w409:bool)
        n263 = Select(t=T23."Disabled and Grayed Out" ("Disabled"), s=w409, f=T23."Enabled" ("Disabled")) -> (s? t:f=w406:T23)
        n264 = property on="Compression" class="Slide (strict)"("DisabledEnum"=w406) -> ()  [unwired: 2 in, 2 out]
      }
    }
  }
  n265 = while {
    tunnel: w48 -> [w414]
    i -> [w417]
    stop <- FALSE stop-if-true
    n266 = Wait (ms)(milliseconds to wait=u32 100) -> ()  [unwired: 1 out]
    n267 = case shown="\"Playback\"" "Rec Mode" {
      tunnel: w417 -> [_ _ w432]
      tunnel: [u32 2829099 ("Base Color") u32 11141120 ("Target Color") w421] -> w413
      frame "Stop", Default {
        # "Reset the color, extra updates don't cost much"
      }
      frame "Record" {
      }
      frame "Playback" {
        # "Playback"
        n268 = Quotient & Remainder(x=w432, y=u32 50 ("milliseconds to wait")) -> (x-y*floor(x/y)=w428:u32)  [unwired: 1 out]
        n269 = Divide(x=w428, y=u32 50 ("milliseconds to wait")) -> (x/y=w425:dbl)
        n270 = Multiply(x=6.283185307179586, y=w425) -> (x*y=w430:dbl)
        n271 = Sine(x=w430) -> (sin(x)=w429:dbl)
        n272 = Absolute Value(x=w429) -> (abs(x)=w422:dbl)
        n273 = call "Interpolate RGB Color.vi"("Proportion"=w422, "Target Color"=u32 30976, "Base Color"=u32 2829099) -> ("Result Color"=w421:u32)  [unwired: 8 in]
      }
    }
    n274 = property class="Pane"(reference=w414, "PaneColor"=w413) -> ()  [unwired: 1 in, 2 out]
  }
  n275 = TCP Create Listener(10:u16 1741 ("timeout ms (25000)")) -> (3:w11:refnum<k5>)  [unwired: 4 in, 2 out]
  n276 = while {
    tunnel: w11 -> [w434]
    stop <- FALSE stop-if-true
    n277 = TCP Wait On Listener(11:w434) -> (4:w433:refnum<k5>)  [unwired: 3 in, 4 out]
    n278 = local write "TCP"(w433) -> ()
  }
  n279 = property on="On/Off" class="Bool (strict)"("Visible"=w16) -> ()  [unwired: 2 in, 2 out]
  n280 = property on="Motor" class="Clust (strict)"("Visible"=w16) -> ()  [unwired: 2 in, 2 out]
  n281 = property on="Progress" class="Clust (strict)"("Visible"=w16) -> ()  [unwired: 2 in, 2 out]
  n282 = property on="Test Ring" class="Ring (strict)"("Visible"=w16) -> ()  [unwired: 2 in, 2 out]
  n283 = property on="Rev/Fwd" class="Clust (strict)"("Visible"=w16) -> ()  [unwired: 2 in, 2 out]
  n284 = property on="Camera Settings" class="Clust (strict)"("Visible"=w16) -> ()  [unwired: 2 in, 2 out]
  n285 = local write "DB Camera Config"(w16) -> ()
  n286 = global write "WPI_DashboardLogging Global.vi" "Recording"(w42) -> ()
  n287 = local write "Rec Mode"(w42) -> ()
  n288 = Build Array("Desired Arm Speed", "Drive Speed", "Desired Stop Distance", "Desired Arm Stop", "Slidewheel Speed", "Close Arm Time") -> (w5:dbl[])
  n289 = call-poly <vilib>:"SD Write Value.vi"("String"="Auto Mode", "Name"="Autonomous Mode") -> ()  [unwired: 8 in, 2 out]
  n290 = call-poly <vilib>:"SD Write Value.vi"("Numeric Array"=w5, "Name"="Autonomous Parameters") -> ()  [unwired: 8 in, 2 out]
